vi "Read Log Folder.vi"(8 "error in (no error)":errorcluster, 11 "Robot Event Local Log in":refnum<class "Robot Event Local Log.lvclass">) -> (0 "error out":errorcluster, 2 "Log Folder":path, 3 "Robot Event Local Log out":refnum<class "Robot Event Local Log.lvclass">)   [LabVIEW 2019, in "Robot Event Local Log.lvclass"]
uses:
  Robot Event Local Log.lvclass
  Robot Event Local Log.lvclass/Robot Event Local Log.ctl
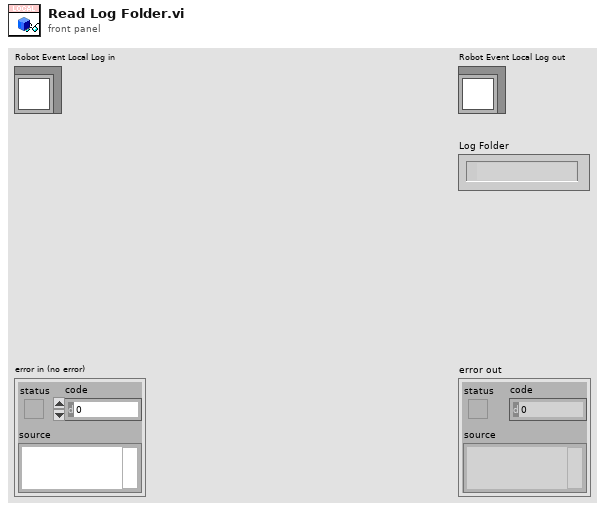
[diagram p1: front panel]
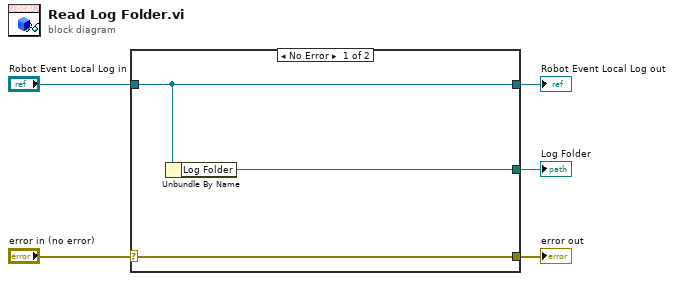
[diagram p0: block diagram]
diagram:
  n1 = case shown="No Error" "error in (no error)" {
    selector: "error in (no error)" -> [w8 w9]
    tunnel: [w8 w9] -> w4
    tunnel: [w7 w10] -> w2
    tunnel: "Robot Event Local Log in" -> [w7 w10]
    tunnel: [w6 _] -> w1
    frame No Error {
      n2 = Unbundle By Name(w7) -> ("Log Folder"=w6:path)
    }
    frame Error {
    }
  }
  "error out" <- w4
  "Robot Event Local Log out" <- w2
  "Log Folder" <- w1
